vi "Check Polarity.vi"(11 "Input Hydra Values":string) -> (1 "Resistance":dbl, 3 "Polarity":dbl, 4 "error out":errorcluster)   [LabVIEW 2020, in "FBN_LATM.lvlib"]
uses:
  FBN_LATM.lvlib
  <vilib>/regexp/Match Regular Expression.xnode
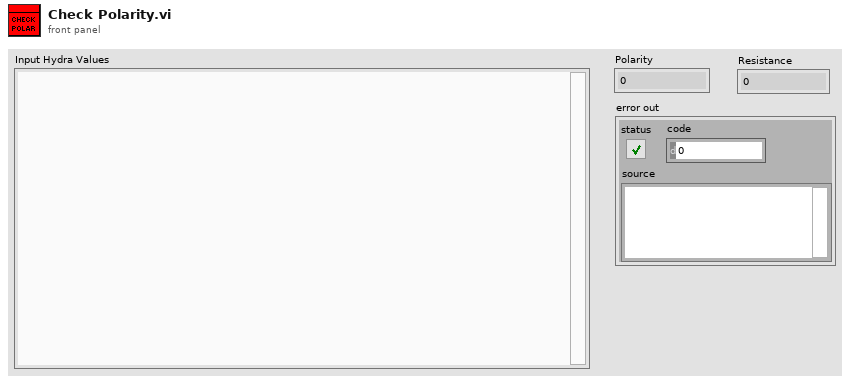
[diagram p1: front panel]
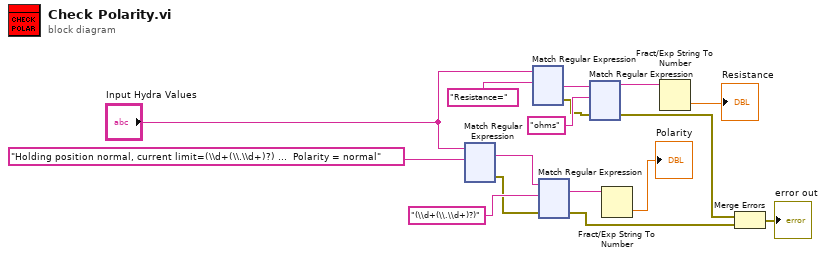
[diagram p0: block diagram]
diagram:
  n1 = xnode "Match Regular Expression"("input string"="Input Hydra Values", "regular expression"="Holding position normal, current limit=(\\d+(\\.\\d+)?) ...  Polarity = normal") -> ("whole match"=w2:string, "error out"=w6:errorcluster)  [unwired: 4 in, 3 out]
  n2 = xnode "Match Regular Expression"("input string"="Input Hydra Values", "regular expression"="Resistance=") -> ("after match"=w13:string, "error out"=w7:errorcluster)  [unwired: 4 in, 3 out]
  n3 = xnode "Match Regular Expression"("input string"=w2, "regular expression"="(\\d+(\\.\\d+)?)", "error in"=w6) -> ("whole match"=w1:string, "error out"=w4:errorcluster)  [unwired: 3 in, 3 out]
  n4 = xnode "Match Regular Expression"("input string"=w13, "regular expression"="ohms", "error in"=w7) -> ("before match"=w10:string, "error out"=w5:errorcluster)  [unwired: 3 in, 3 out]
  n5 = Fract/Exp String To Number(string=w1) -> (number=→"Polarity":dbl)  [unwired: 3 in, 1 out]
  n6 = Fract/Exp String To Number(string=w10) -> (number=→"Resistance":dbl)  [unwired: 3 in, 1 out]
  n7 = Merge Errors(w5, w4) -> (→"error out":errorcluster)
